vi "AlliGator Build Python Plugin Parameter Map.vi"(8 "error in (no error)":errorcluster, 9 "Parameter_Map_Data":T1, 10 "Function Display Name":string, 11 "[Map Set Names] in":string[](array[string])) -> (0 "error out":errorcluster, 1 "New Parameter Names":string[](array[string]), 2 "Parameter Map out":T3, 3 "[Map Set Names] out":string[](array[string]), 4 "Message":string)   [LabVIEW 2021, in "AlliGator Python Plugins.lvlib"]
uses:
  AlliGator Python Plugins.lvlib
  Decay Fit Parameter Map/AlliGator Parameter Maps Data.ctl
  API v1.1/AlliGator Python Plugin Parameter Map Data v1.1.ctl
  Image/Image Point.ctl
  Decay Fit Parameter Map/AlliGator Decay Fit Parameter Map.lvlib
  Strings/Strings.lvlib
  Image/Image.lvlib
panel:
  # "see the License on the block diagram (Ctrl+E or Window:Show Block Diagram)"
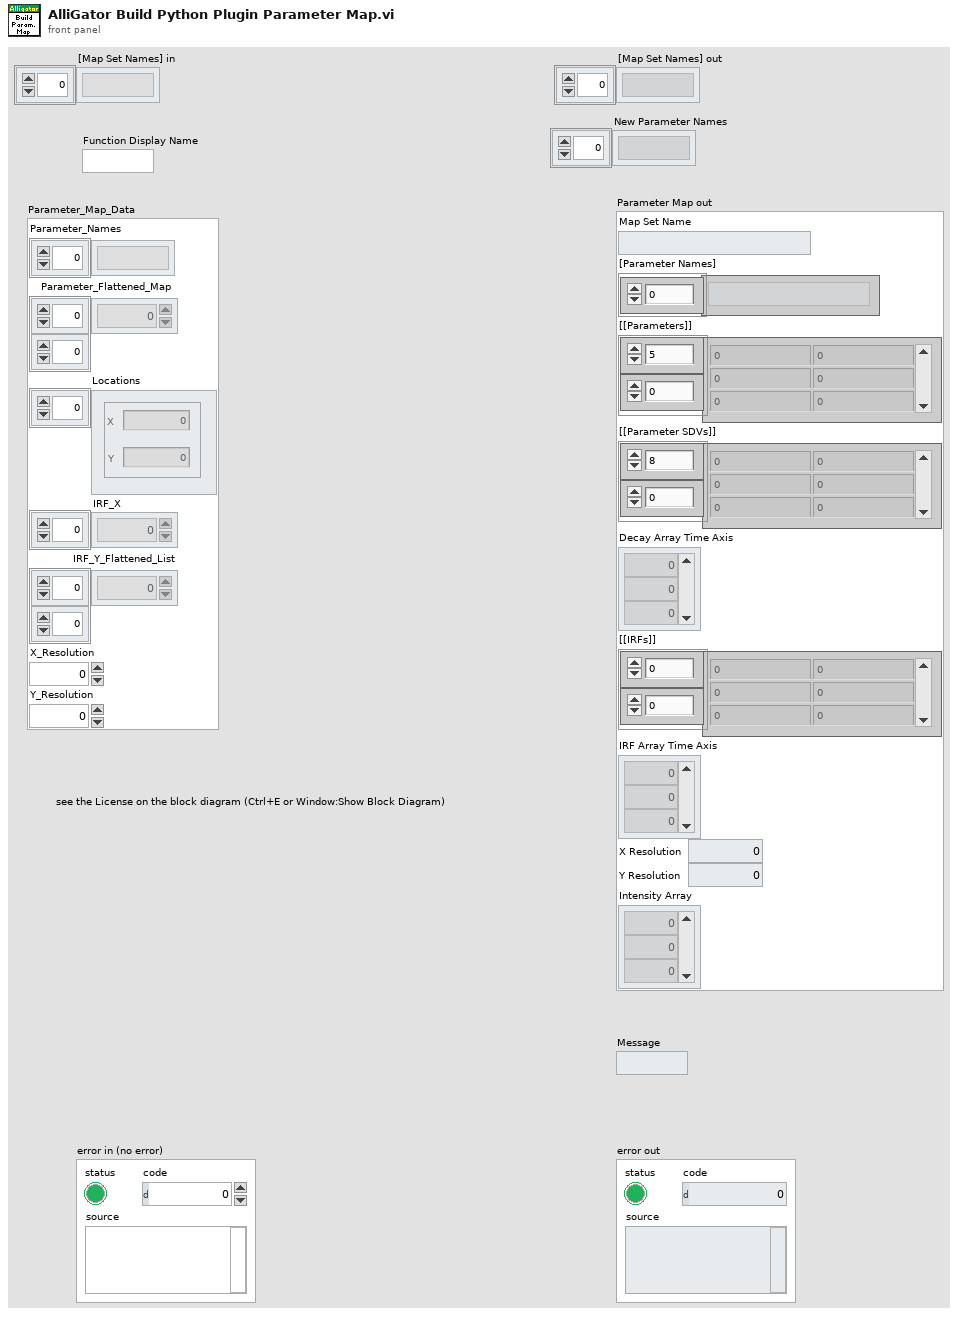
[diagram p1: front panel]
types:
  T1 = typedef "AlliGator Python Plugins.lvlib/AlliGator Python Plugin Parameter Map Data v1.1.ctl" = cluster{"Parameter_Names":string[], "Parameter_Flattened_Map":dbl[][], "Locations":T2[], "IRF_X":dbl[], "IRF_Y_Flattened_List":dbl[][], "X_Resolution":i32, "Y_Resolution":i32}
  T2 = typedef "Image.lvlib/Image Point.ctl" = cluster{"X":i32, "Y":i32}
  T3 = typedef "AlliGator Decay Fit Parameter Map.lvlib/AlliGator Parameter Maps Data.ctl" = cluster{"Map Set Name":string, "[Parameter Names]":string[], "[[Parameters]]":dbl[][], "[[Parameter SDVs]]":dbl[][], "Decay Array Time Axis":dbl[], "[[IRFs]]":dbl[][], "IRF Array Time Axis":dbl[], "X Resolution":i32, "Y Resolution":i32, "Intensity Array":dbl[]}
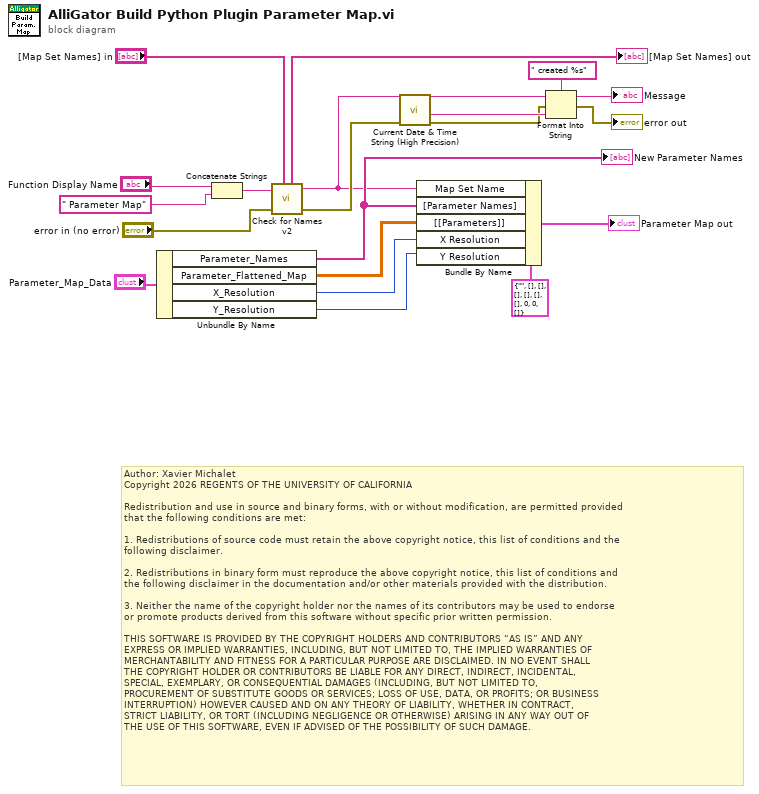
[diagram p0: block diagram]
diagram:
  # "Author: Xavier Michalet\nCopyright 2026 REGENTS OF THE UNIVERSITY OF CALIFORNIA\n\nRedistribution and use in source and binary forms, with or without modification, are permitted provided\nthat the following conditions are met:\n\n1. Redistributions of source code must retain the above copyright notice, this list of conditions and the\nfollowing disclaimer.\n\n2. Redistributions in binary form must reproduce the above copyright notice, this list of conditions and\nthe following disclaimer in the documentation and/or other materials provided with the distribution.\n\n3. Neither the name of the copyright holder nor the names of its contributors may be used to endorse \nor promote products derived from this software without specific prior written permission.\n\nTHIS SOFTWARE IS PROVIDED BY THE COPYRIGHT HOLDERS AND CONTRIBUTORS “AS IS” AND ANY \nEXPRESS OR IMPLIED WARRANTIES, INCLUDING, BUT NOT LIMITED TO, THE IMPLIED WARRANTIES OF\nMERCHANTABILITY AND FITNESS FOR A PARTICULAR PURPOSE ARE DISCLAIMED. IN NO EVENT SHALL\nTHE COPYRIGHT HOLDER OR CONTRIBUTORS BE LIABLE FOR ANY DIRECT, INDIRECT, INCIDENTAL, \nSPECIAL, EXEMPLARY, OR CONSEQUENTIAL DAMAGES (INCLUDING, BUT NOT LIMITED TO, \nPROCUREMENT OF SUBSTITUTE GOODS OR SERVICES; LOSS OF USE, DATA, OR PROFITS; OR BUSINESS\nINTERRUPTION) HOWEVER CAUSED AND ON ANY THEORY OF LIABILITY, WHETHER IN CONTRACT, \nSTRICT LIABILITY, OR TORT (INCLUDING NEGLIGENCE OR OTHERWISE) ARISING IN ANY WAY OUT OF\nTHE USE OF THIS SOFTWARE, EVEN IF ADVISED OF THE POSSIBILITY OF SUCH DAMAGE."
  n1 = Unbundle By Name("Parameter_Map_Data") -> ("Parameter_Names"=w5:string[], "Parameter_Flattened_Map"=w4:dbl[][], "X_Resolution"=w3:i32, "Y_Resolution"=w2:i32)
  "New Parameter Names" <- w5
  n2 = Concatenate Strings("Function Display Name", " Parameter Map" ("string")) -> (w18:string)
  n3 = call "Check for Names v2.vi"("New Name"=w18, "Name List"="[Map Set Names] in", "Error In"="error in (no error)") -> ("New Name List"=→"[Map Set Names] out":string[], "New Name"=w1:string, "Error Out"=w8:errorcluster)  [unwired: 3 in, 1 out]
  n4 = call "Current Date & Time String (High Precision).vi"("Error In"=w8) -> ("Error Out"=w7:errorcluster, "on <Date> at <Time>"=w9:string)  [unwired: 7 in, 2 out]
  n5 = Bundle By Name(cluster=T3 {"Map Set Name"="", "[Parameter Names]"=[], "[[Parameters]]"=[], "[[Parameter SDVs]]"=[], "Decay Array Time Axis"=[], "[[IRFs]]"=[], "IRF Array Time Axis"=[], "X Resolution"=0, "Y Resolution"=0, "Intensity Array"=[]} ("[Parameter Maps]"), "Map Set Name"=w1, "[Parameter Names]"=w5, "[[Parameters]]"=w4, "X Resolution"=w3, "Y Resolution"=w2) -> (→"Parameter Map out":T3)
  n6 = Format Into String(format string=" created %s", initial string=w1, error in=w7, w9) -> (resulting string=→"Message":string, error out=→"error out":errorcluster)
